vi "Unit Test Preserve wired non-serialized data (Same) True.vi"() -> ()   [LabVIEW 2019, in "Sports Unit Tests.lvclass"]
uses:
  Sports Unit Tests.lvclass
  <vilib>/addons/_JKI Toolkits/Caraya/classes/Assert/Assert.lvclass
  Classes/Adam Sandler/Adam Sandler.lvclass
  <vilib>/addons/_JKI Toolkits/Caraya/classes/Assert/Assert Equal Value_Variant.vi
  <vilib>/addons/_JKI Toolkits/Caraya/classes/Assert/Assert Not Error.vi
  <userlib>/Blue Origin/BlueSerialization/BlueSerializer/DeserializeMutationOptions.ctl
  <userlib>/Blue Origin/BlueSerialization/BlueSerializer/BlueSerializer.lvclass
  <userlib>/Blue Origin/BlueSerialization/BlueSerializer/DeserializeSlicingOptions.ctl
  <userlib>/Blue Origin/BlueSerialization/BlueSerializer/DeserializeOptions.ctl
  <userlib>/Blue Origin/BlueSerialization/BlueSerializer/DeserializePreservationOptions.ctl
  <userlib>/Blue Origin/BlueSerialization/BlueSerializer/PreserveNonWiredDataOption.ctl
panel:
  out "Table":string[][](table)
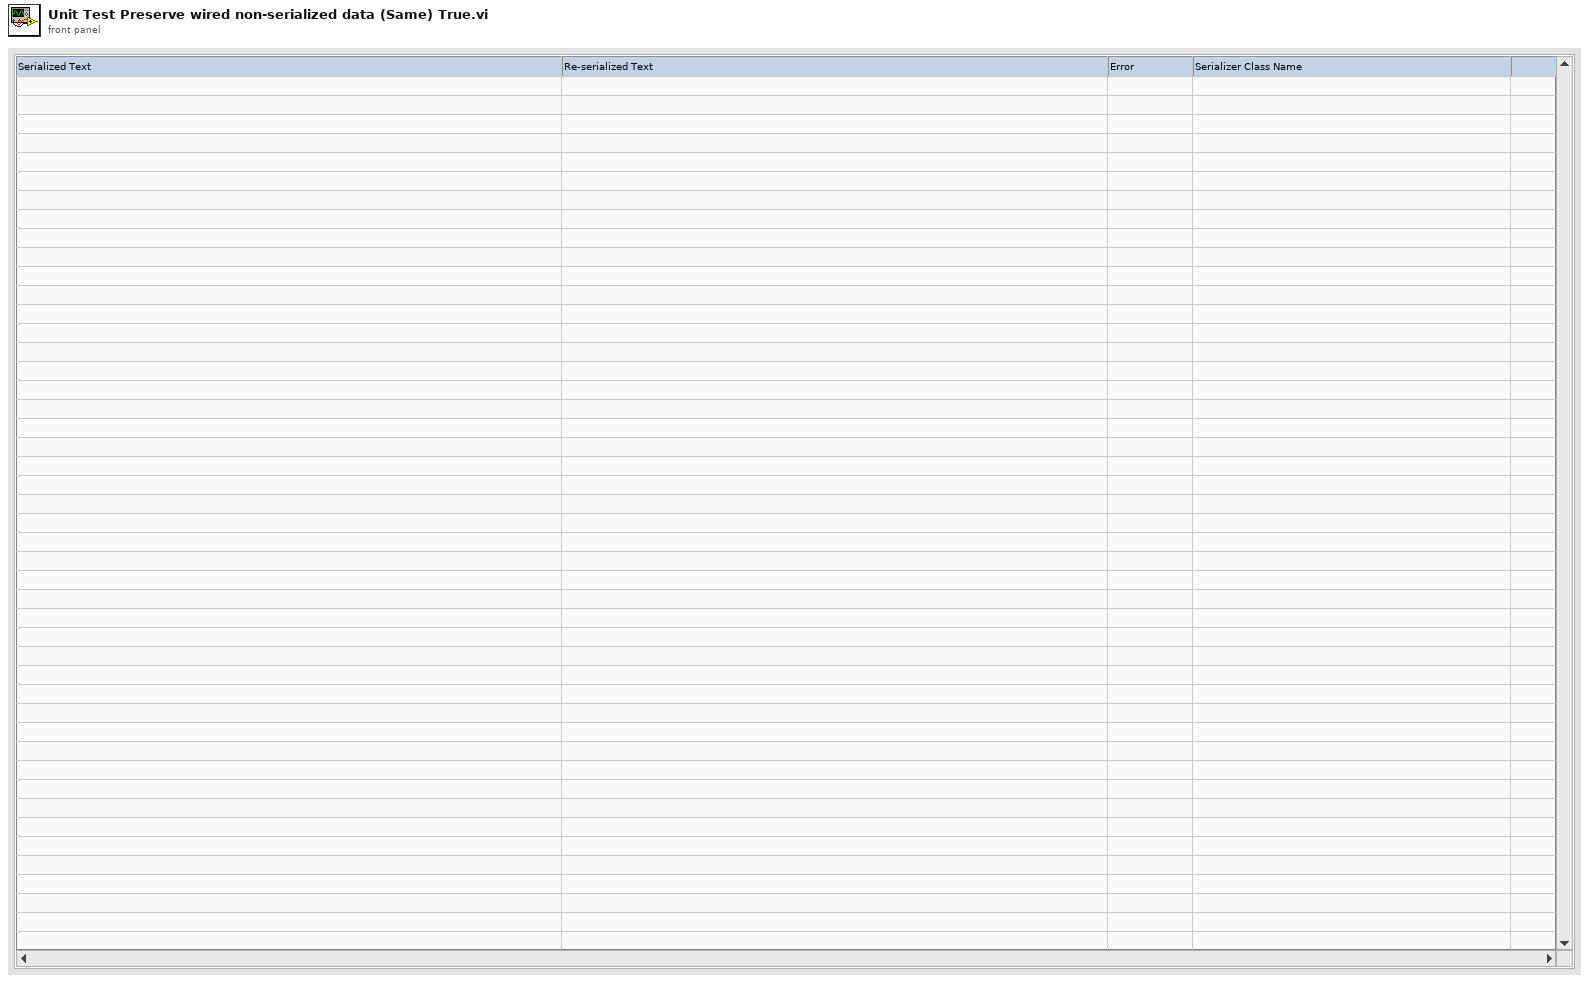
[diagram p1: front panel]
types:
  T1 = typedef "BlueSerialization.lvlib/BlueSerializer.lvclass/PreserveNonWiredDataOption.ctl" = enum16{"Don't preserve", "Preserve (error on less-specific wired types)", "Preserve (except on less-specific wired types)"}
  T2 = typedef "BlueSerialization.lvlib/BlueSerializer.lvclass/DeserializeOptions.ctl" = cluster{"deserialize non-BlueSerializable objects from hex?":bool, "expand objects on type conflict?":bool, "Slicing":T3, "Mutation Options":T4, "Preservation Options":T5}
  T3 = typedef "BlueSerialization.lvlib/BlueSerializer.lvclass/DeserializeSlicingOptions.ctl" = cluster{"slice flattened object data on error?":bool, "sliceable class names":string[]}
  T4 = typedef "BlueSerialization.lvlib/BlueSerializer.lvclass/DeserializeMutationOptions.ctl" = cluster{"error on inserted parent levels?":bool, "\terror on obsolete parent levels?":bool}
  T5 = typedef "BlueSerialization.lvlib/BlueSerializer.lvclass/DeserializePreservationOptions.ctl" = cluster{"Preserve wired serialized data?":bool, "Preserve wired non-serialized data":T1}
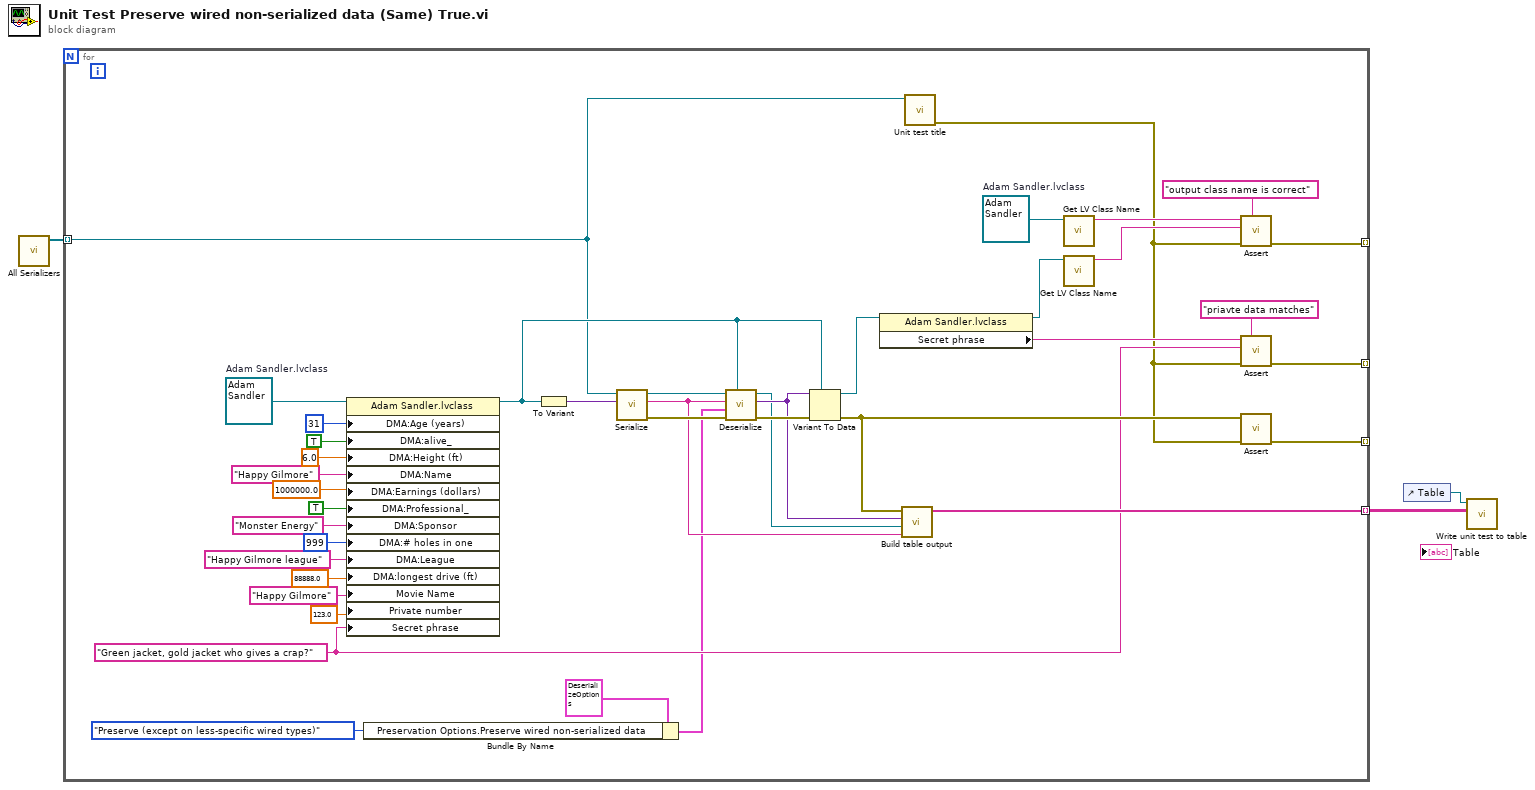
[diagram p0: block diagram]
diagram:
  n1 = call "All Serializers.vi"() -> ("All serializers"=w2:refnum<class "BlueSerializer.lvclass">[])  [unwired: 11 in]
  n2 = for {
    tunnel: w2 -> [w7] mode=indexing
    tunnel: [w29] -> _ mode=indexing
    tunnel: [w28] -> _ mode=indexing
    tunnel: [w23] -> w1 mode=indexing
    tunnel: [w9] -> _ mode=indexing
    w16 = refnum<class "Adam Sandler.lvclass"> refnum  # Adam Sandler.lvclass
    w11 = "Green jacket, gold jacket who gives a crap?" ("Secret phrase")
    w22 = refnum<class "Adam Sandler.lvclass"> refnum  # Adam Sandler.lvclass
    n3 = property on="Property Node" class="Adam Sandler.lvclass"(reference=w22, "DMA:Age (years)"=u16 31 ("Age (years)"), "DMA:alive_"=TRUE ("alive_"), "DMA:Height (ft)"=6.0 ("Height (ft)"), "DMA:Name"="Happy Gilmore" ("Name"), "DMA:Earnings (dollars)"=1000000.0 ("Earnings (dollars)"), "DMA:Professional_"=TRUE ("Professional_"), "DMA:Sponsor"="Monster Energy" ("Sponsor"), "DMA:# holes in one"=999 ("# holes in one"), "DMA:League"="Happy Gilmore league" ("League"), "DMA:longest drive (ft)"=88888.0 ("longest drive (ft)"), "Movie Name"="Happy Gilmore", "Private number"=123.0, "Secret phrase"=w11) -> (reference out=w8:refnum<class "Adam Sandler.lvclass">)  [unwired: 1 in, 1 out]
    n4 = Bundle By Name(cluster=T2 {"deserialize non-BlueSerializable objects from hex?"=FALSE, "expand objects on type conflict?"=FALSE, "Slicing"={"slice flattened object data on error?"=FALSE, "sliceable class names"=[]}, "Mutation Options"={"error on inserted parent levels?"=FALSE, "\terror on obsolete parent levels?"=FALSE}, "Preservation Options"={"Preserve wired serialized data?"=FALSE, "Preserve wired non-serialized data"=enum."Don't preserve"}} ("Deserialize Options"), "Preservation Options.Preserve wired non-serialized data"=PreserveNonWiredDataOption."Preserve (except on less-specific wired types)") -> (w5:T2)
    n5 = To Variant(anything=w8) -> (Variant=w41:variant)
    n6 = call <userlib>:"Serialize.vi"("Anything"=w41, "BlueSerializer in"=w7) -> ("error out"=w43:errorcluster, "Serialized Text"=w24:string, "BlueSerializer out"=w42:refnum<class "BlueSerializer.lvclass">)  [unwired: 7 in]
    n7 = call <userlib>:"Deserialize.vi"("Anything"=w8, "error in (no error)"=w43, "Deserialize Options"=w5, "Serialized Text"=w24, "BlueSerializer in"=w42) -> ("error out"=w40:errorcluster, "Variant"=w26:variant, "BlueSerializer out"=w25:refnum<class "BlueSerializer.lvclass">)  [unwired: 4 in]
    n8 = Variant To Data(error in=w40, type=w8, Variant=w26) -> (data=w14:refnum<class "Adam Sandler.lvclass">, error out=w27:errorcluster)
    n9 = property class="Adam Sandler.lvclass"(reference=w14) -> (reference out=w13:refnum<class "Adam Sandler.lvclass">, "Secret phrase"=w12:string)  [unwired: 1 in, 1 out]
    n10 = call "Build table output.vi"("serialized text"=w24, "BlueSerializer in"=w25, "deserialized variant"=w26, "variant to data error"=w27) -> ("table output"=w23:string[])  [unwired: 7 in]
    n11 = call "Unit test title.vi"("serializer"=w7) -> ("error out"=w10:errorcluster)  [unwired: 9 in, 1 out]
    n12 = call <vilib>:"Get LV Class Name.vi"("object"=w16) -> ("class name"=w39:string)  [unwired: 9 in, 1 out]
    n13 = call <vilib>:"Get LV Class Name.vi"("object"=w13) -> ("class name"=w38:string)  [unwired: 9 in, 1 out]
    n14 = call-poly <vilib>:"Assert.vi"("Label"="output class name is correct", "error in (no error)"=w10, "Y"=w38, "X"=w39) -> ("error out"=w28:errorcluster)  [unwired: 7 in]
    n15 = call-poly <vilib>:"Assert.vi"("Label"="priavte data matches", "error in (no error)"=w10, "Y"=w11, "X"=w12) -> ("error out"=w9:errorcluster)  [unwired: 7 in]
    n16 = call-poly <vilib>:"Assert.vi"("error in (no error)"=w10, "Not Error?"=w27) -> ("error out"=w29:errorcluster)  [unwired: 9 in]
  }
  n17 = control-ref of="Table"() -> (w3:refnum<vi>)
  n18 = call "Write unit test to table.vi"("Table"=w1, "Table ref in"=w3) -> ()  [unwired: 9 in, 1 out]
